vi "backproject-normalise.vi"(8 "Ctl Refnum":refnum<vi>, 9 "Image Properties":T1, 10 "Backproject Input":T2, 11 "Queue in":refnum<queue>) -> (0 "queue out":refnum<queue>, 1 "Normalisation":i32[](array[numeric]), 2 "Array":sgl[](array[numeric]), 3 "Intermediate":sgl[](array[numeric]))   [LabVIEW 2013]
uses:
  backproject_input.ctl
  tags_cluster.ctl
panel:
  out "Current summing work unit #":i32
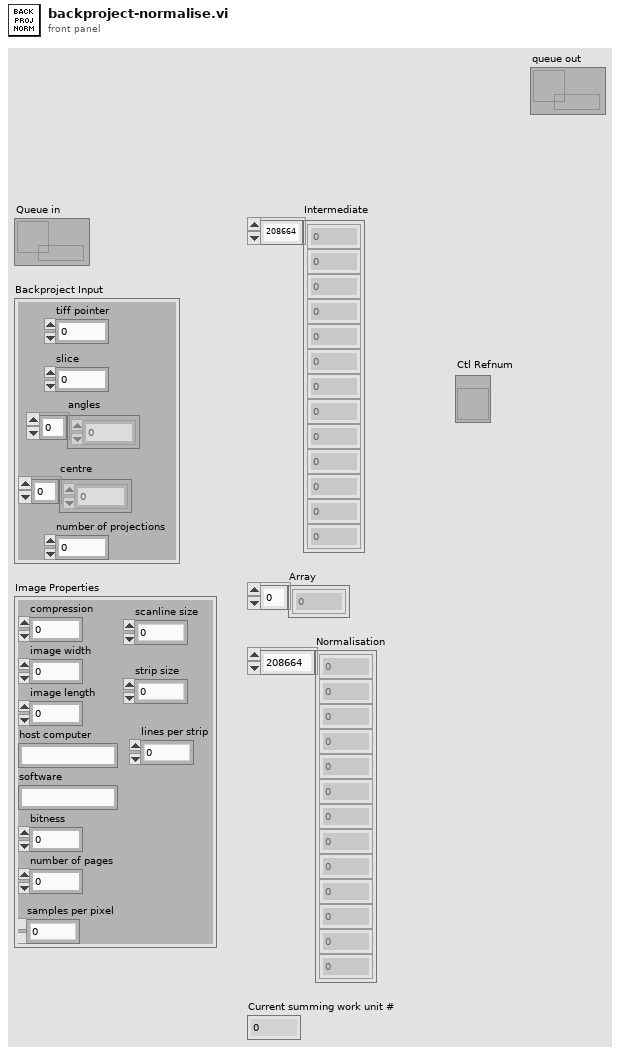
[diagram p1: front panel]
types:
  T1 = typedef "tags_cluster.ctl" = cluster{"compression":i32, "image width":i32, "image length":i32, "host computer":string, "software":string, "bitness":i32, "number of pages":i32, "samples per pixel":i32, "scanline size":i32, "strip size":i32, "lines per strip":i32}
  T2 = typedef "backproject_input.ctl" = cluster{"tiff pointer":i64, "slice":u32, "angles":dbl[], "centre":i32[], "number of projections":u32}
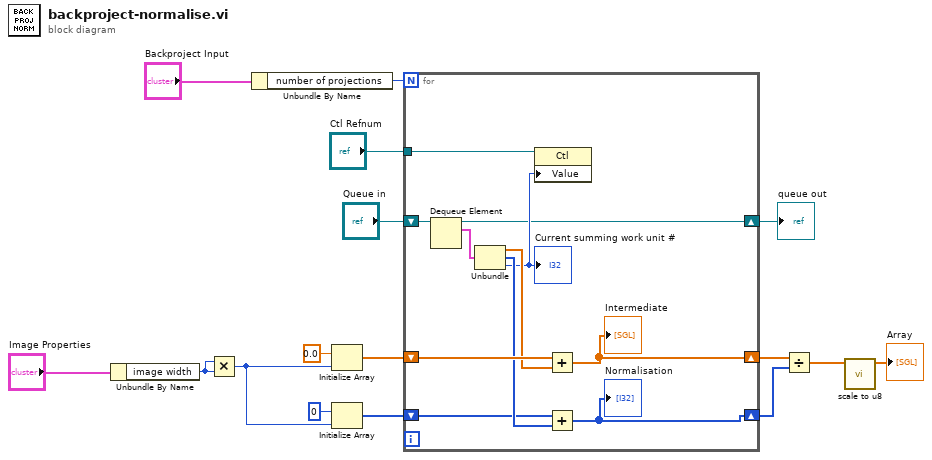
[diagram p0: block diagram]
diagram:
  n1 = Unbundle By Name("Image Properties") -> ("image width"=w6:i32)
  n2 = Multiply(x=w6, y=w6) -> (x*y=w9:i32)
  n3 = Unbundle By Name("Backproject Input") -> ("number of projections"=w16:u32)
  n4 = Initialize Array(sgl 0.0 ("element"), w9) -> (w7:sgl[])
  n5 = Initialize Array(0 ("element"), w9) -> (w10:i32[])
  n6 = for {
    N: w16 -> [_]
    shift-right: [w23] -> w11
    shift-left: w7 -> [w25]
    shift-right: [w20] -> w12
    shift-left: w10 -> [w21]
    tunnel: "Ctl Refnum" -> [w18]
    shift-right: [w17] -> w1
    shift-left: "Queue in" -> [w27]
    n7 = Dequeue Element(queue=w27) -> (queue out=w17:refnum<queue>, element=w26:cluster{sgl[], i32[], i32})  [unwired: 2 in, 2 out]
    n8 = Unbundle(w26) -> (w24:sgl[], w22:i32[], w19:i32)
    "Current summing work unit #" <- w19
    n9 = property class="Ctl"(reference=w18, "Value"=w19) -> ()  [unwired: 1 in, 2 out]
    n10 = Add(x=w25, y=w24) -> (x+y=w23:sgl[])
    "Intermediate" <- w23
    n11 = Add(x=w21, y=w22) -> (x+y=w20:i32[])
    "Normalisation" <- w20
  }
  "queue out" <- w1
  n12 = Divide(x=w11, y=w12) -> (x/y=w3:sgl[])
  n13 = call "scale to u8.vi"("Input"=w3) -> ("Output"=→"Array":sgl[])  [unwired: 10 in]
